vi "Simulador.vi"() -> ()   [LabVIEW 2014]
uses:
  <vilib>/imath/engines/lvmath/Plug In/_Char/NIMS_CH_character datatype.ctl
  <vilib>/imath/engines/lvmath2/RunTimeEngine/Managers/WorkSpace/UID Generator.vi
  <vilib>/imath/engines/lvmath2/RunTimeEngine/BuiltInFunctions/var/NIMS_var(GV,RV).vi
  <instcachedir>/0/NIMS_var(GV,RV)_4069E0180F614BA3BA7EF465AF0C1F39.lvgen/NIMS_var(GV,RV)_4069E0180F614BA3BA7EF465AF0C1F39_001.vi
  <vilib>/imath/engines/lvmath2/RunTimeEngine/RunTimeType/NIMS_RunTimeType_From StrictType (excl LVString).vi
  <instcachedir>/0/NIMS_RunTimeType_From StrictType (excl LVString)_15A5391EEA9C4AACB9955AC755B83D29.lvgen/NIMS_RunTimeType_From StrictType (excl LVString)_15A5391EEA9C4AACB9955AC755B83D29_000.vi
  <vilib>/imath/engines/lvmath2/RunTimeEngine/ErrorHandling/NIMS_Error From Error Code.vi
  <vilib>/imath/engines/lvmath2/RunTimeEngine/LocalVariableDefStatement/MC_LocalVariableDefStatement_Display.vi
  <vilib>/imath/engines/lvmath/Plug In/_Char/NIMS_CH_Character 1D to U8 1D.vi
  <vilib>/imath/engines/lvmath2/RunTimeEngine/Managers/SymbolTable/Clear UID.vi
  <vilib>/imath/engines/lvmath2/RunTimeEngine/NodeEndStatement/NIMS_NodeEndStatement_Output.vi
  <instcachedir>/0/NIMS_NodeEndStatement_Output_53EC0D466D134D7ABD903AC30B43404B.lvgen/NIMS_NodeEndStatement_Output_53EC0D466D134D7ABD903AC30B43404B_011.vi
  <vilib>/imath/engines/lvmath2/RunTimeEngine/ErrorHandling/NIMS_Finalize Error.vi
  <vilib>/imath/engines/lvmath2/RunTimeEngine/Managers/SymbolTable/NIMS_WorkSpace.lvlib
panel:
  out "Numeric":dbl
  out "Tank":dbl(slide) scale=0.0..30.0
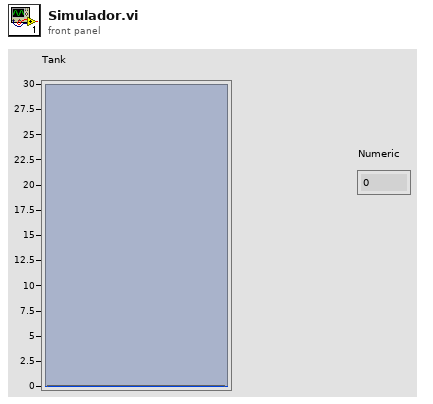
[diagram p1: front panel]
types:
  T1 = typedef "NIMS_CH_character datatype.ctl" = cluster{"Numeric":u8}
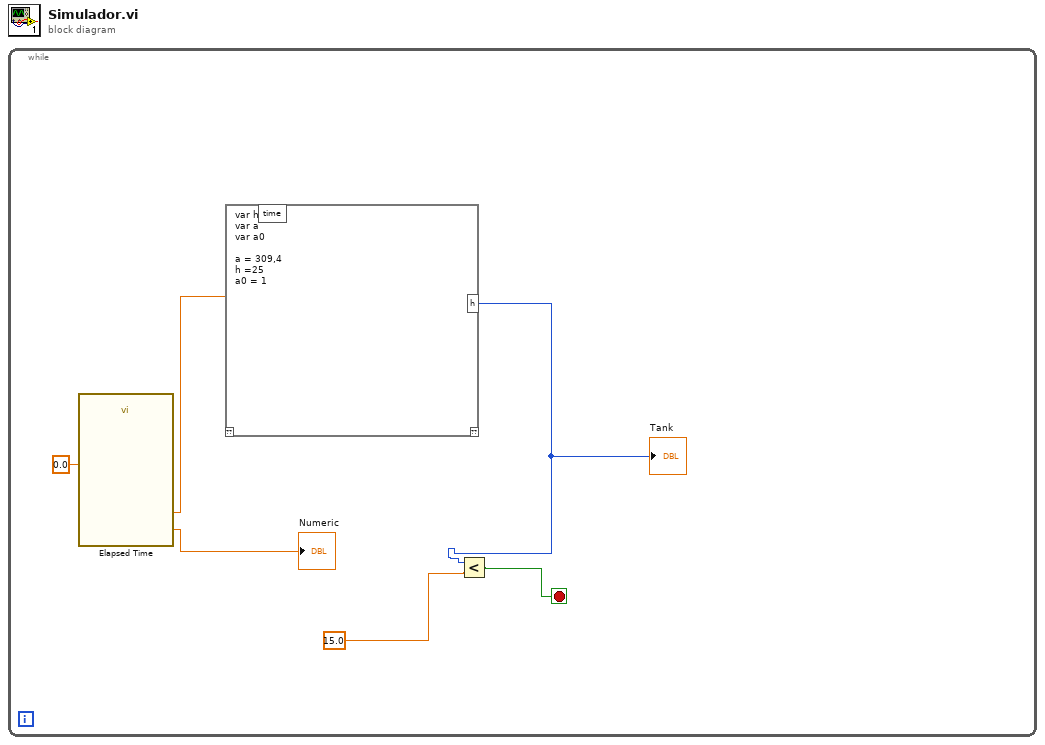
[diagram p0: block diagram]
diagram:
  n1 = while {
    stop <- w2 stop-if-true
    n2 = call "Elapsed Time"("Set Start Time (s)"=0.0) -> ("Present (s)"=→"Numeric":dbl, "Elapsed Time (s)"=w5:dbl)  [unwired: 11 in, 6 out]
    n3 = mathscript code="var h \nvar a\nvar a0\n\na = 309,4\nh =25\na0 = 1"("time"=w5) -> ("h"=w4:i32)  [unwired: 1 in, 1 out]
    "Tank" <- w4
    n4 = Less?(x=w4, y=15.0 ("Set Start Time (s)")) -> (x < y?=w2:bool)
  }
